vi "LogToSyslog.vi"(7 "severity (informational)":i32(ring)=2 items=["Error", "Warning", "Informational"], 10 "error in (no error)":errorcluster, 11 "message":string) -> (2 "error out":errorcluster, 3 "Syslog Message":string)   [LabVIEW 2020, in "Ballard 1553 Shared.lvlib"]
uses:
  Ballard 1553 Shared.lvlib
  <vilib>/Utility/SystemLogging/NI_SystemLogging.lvlib
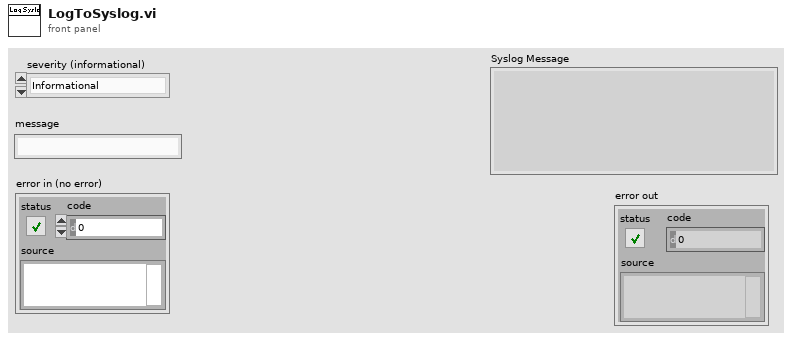
[diagram p1: front panel]
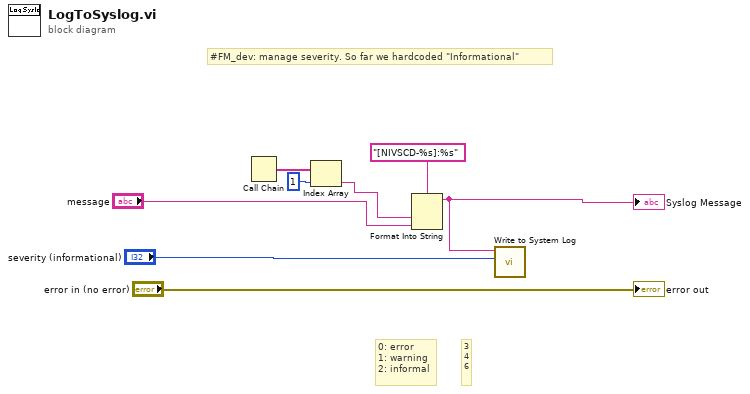
[diagram p0: block diagram]
diagram:
  # "3\n4\n6"
  # "0: error\n1: warning\n2: informal"
  # "#FM_dev: manage severity. So far we hardcoded \"Informational\""
  n1 = Call Chain() -> (call chain=w4:string[])
  n2 = Index Array(array=w4, index=1) -> (element=w1:string)
  n3 = Format Into String(format string="[NIVSCD-%s]:%s", w1, "message") -> (resulting string=w5:string)  [unwired: 2 in, 1 out]
  "Syslog Message" <- w5
  n4 = call <vilib>:"Write to System Log.vi"("severity"="severity (informational)", "message"=w5) -> ()  [unwired: 9 in, 1 out]
  "error out" <- "error in (no error)"
